vi "Drone.vi"() -> ()   [LabVIEW 2009]
uses:
  square.ctl
  Drone data.ctl
panel:
  out "iteration":i32
  in  "Import drones":path[](array[path])
  in  "create drones":T1[](array[typedef])=[{"Current"={"location"={"x"=0, "y"=0}, "checkpoint"=0}, "Checkpoints"=[{"x"=16, "y"=16}, {"x"=0, "y"=0}], "Color"=11145540, "Navigation style"=4}, {"Current"={"location"={"x"=31, "y"=16}, "checkpoint"=0}, "Checkpoints"=[{"x"=16, "y"=16}, {"x"=0, "y"=0}], "Color"=11145540, "Navigation style"=3}]
  in  "walls":path
  in  "stop":bool
  in  "Delay (ms)":u32
  out "map":T2[][](array[typedef])
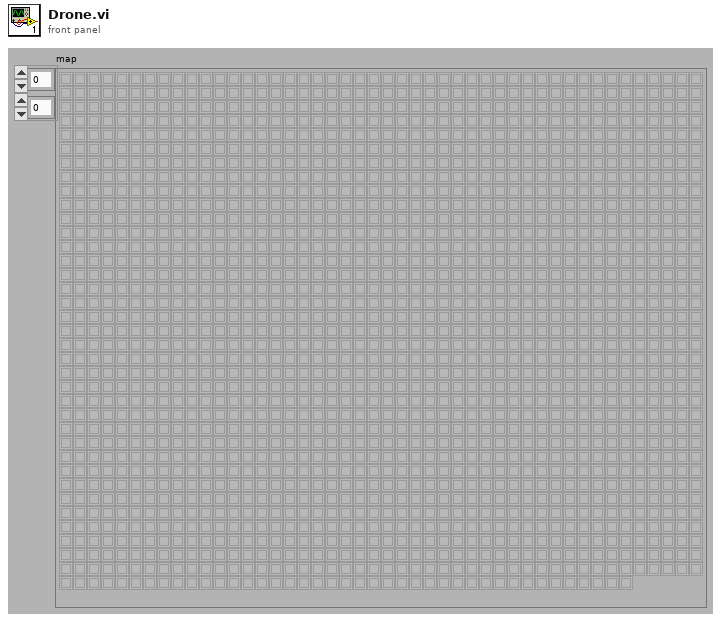
[diagram p1: front panel]
types:
  T1 = typedef "Drone data.ctl" = cluster{"Current":cluster{"location":cluster{"x":i16, "y":i16}, "checkpoint":i32}, "Checkpoints":cluster{"x":i16, "y":i16}[], "Color":u32, "Navigation style":i32}
  T2 = typedef "square.ctl" = u8
  T3 = typedef "direction.ctl" = i8
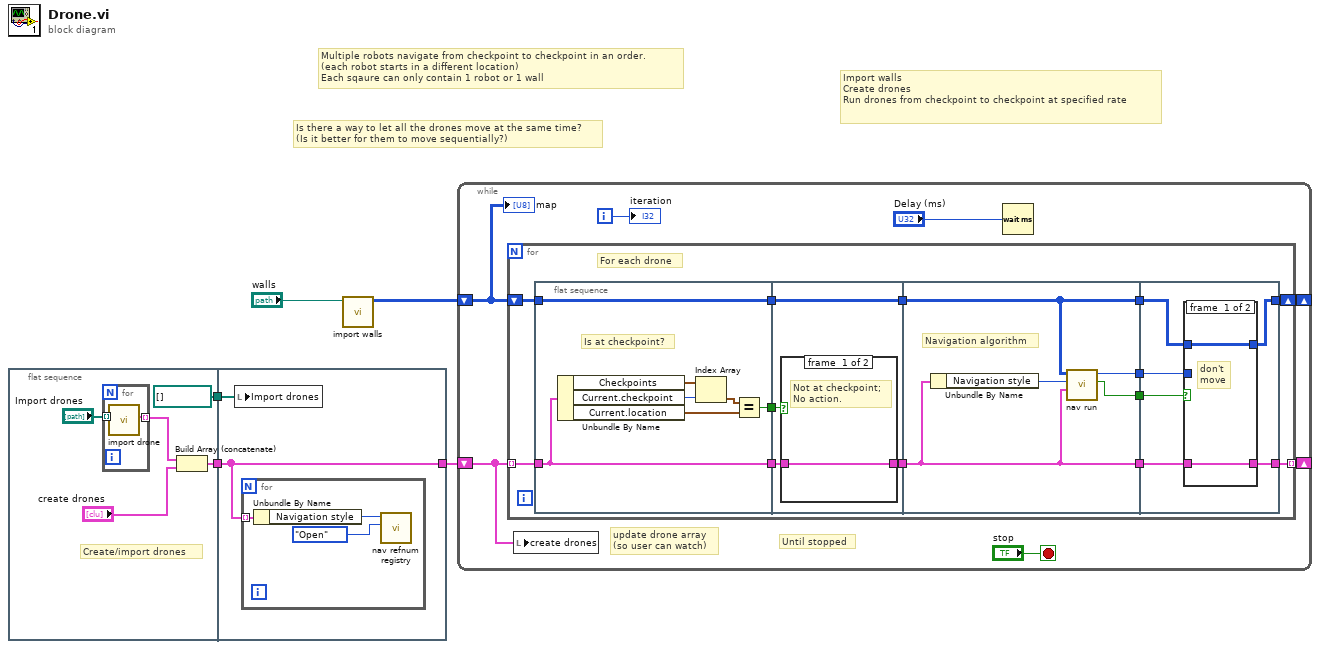
[diagram p0: block diagram]
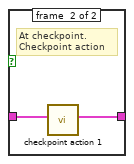
[diagram p2: hidden frame]
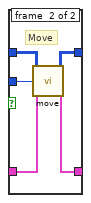
[diagram p3: hidden frame]
diagram:
  # "Is there a way to let all the drones move at the same time?\n(Is it better for them to move sequentially?)"
  # "Import walls\nCreate drones\nRun drones from checkpoint to checkpoint at specified rate"
  # "Multiple robots navigate from checkpoint to checkpoint in an order.\n(each robot starts in a different location)\nEach sqaure can only contain 1 robot or 1 wall"
  n1 = flat-sequence {
    tunnel: [w8] -> w2
    tunnel: [path[] [] ("Import drones")] -> w1
    tunnel: [w13] -> w3
    tunnel: w2 -> [w13]
    tunnel: w1 -> [w14]
    frame #0 {
      # "Create/import drones"
      n2 = for {
        tunnel: [w12] -> w10 mode=indexing
        tunnel: "Import drones" -> [w11] mode=indexing
        n3 = call "import drone.vi"("drone filepath"=w11) -> ("Drone"=w12:T1)  [unwired: 9 in, 1 out]
      }
      n4 = Build Array (concatenate)(w10, "create drones") -> (w8:T1[])
    }
    frame #1 {
      n5 = local write "Import drones"(w14) -> ()
      n6 = for {
        tunnel: w13 -> [w17] mode=indexing
        n7 = Unbundle By Name(w17) -> ("Navigation style"=w16:i32)
        n8 = call "nav refnum registry.vi"("Action"=enum16{"Open", "Retreive", "Close"}."Open", "nav type"=w16) -> ()  [unwired: 8 in, 2 out]
      }
    }
  }
  n9 = call "import walls.vi"("Picture path"="walls") -> ("walls/field"=w4:T2[][])  [unwired: 10 in]
  n10 = while {
    shift-right: [w24] -> _
    shift-left: w3 -> [w19]
    shift-right: [w23] -> _
    shift-left: w4 -> [w22]
    i -> [w18]
    stop <- "stop" stop-if-true
    # "update drone array\n(so user can watch)"
    # "Until stopped"
    n11 = for {
      tunnel: w19 -> [w36] mode=indexing
      tunnel: [w35] -> w24 mode=indexing
      shift-right: [w30] -> w23
      shift-left: w22 -> [w27]
      # "For each drone"
      n12 = flat-sequence {
        tunnel: [w39] -> w37
        tunnel: w36 -> [w38]
        tunnel: [w38] -> w32
        tunnel: [w44] -> w28
        tunnel: w27 -> [w44]
        tunnel: w37 -> [w48]
        tunnel: [w46] -> w33
        tunnel: w32 -> [w45]
        tunnel: [w47] -> w29
        tunnel: w28 -> [w47]
        tunnel: [w54] -> w34
        tunnel: [w55] -> w31
        tunnel: w29 -> [w55]
        tunnel: w33 -> [w54]
        tunnel: [w53] -> w26
        tunnel: [w52] -> w25
        tunnel: [w60] -> w35
        tunnel: w34 -> [w59]
        tunnel: [w61] -> w30
        tunnel: w31 -> [w62]
        tunnel: w26 -> [w58]
        tunnel: w25 -> [w57]
        frame #0 {
          # "Is at checkpoint?"
          n13 = Unbundle By Name(w38) -> ("Checkpoints"=w42:cluster{"x":i16, "y":i16}[], "Current.checkpoint"=w43:i32, "Current.location"=w40:cluster{"x":i16, "y":i16})
          n14 = Index Array(array=w42, index=w43) -> (element=w41:cluster{"x":i16, "y":i16})
          n15 = Equal?(x=w41, y=w40) -> (x = y?=w39:bool)
        }
        frame #1 {
          n16 = case shown="True" w48 {
            tunnel: [w49 w50] -> w46
            tunnel: w45 -> [w49 w51]
            frame #0 {
              # "Not at checkpoint;\nNo action."
            }
            frame #1 {
              # "At checkpoint.\nCheckpoint action"
              n17 = call "checkpoint action 1.vi"("Drone"=w51) -> ("Drone"=w50:T1)  [unwired: 10 in]
            }
          }
        }
        frame #2 {
          # "Navigation algorithm"
          n18 = Unbundle By Name(w54) -> ("Navigation style"=w56:i32)
          n19 = call "nav run.vi"("Drone"=w54, "nav type"=w56, "Field"=w55) -> ("Move?"=w52:bool, "direction"=w53:T3)  [unwired: 7 in]
        }
        frame #3 {
          n20 = case shown="True" w57 {
            tunnel: w62 -> [w64 w69]
            tunnel: [w64 w67] -> w61
            tunnel: [w63 w66] -> w60
            tunnel: w59 -> [w63 w68]
            tunnel: w58 -> [_ w65]
            frame #0 {
              # "don't\nmove"
            }
            frame #1 {
              # "Move"
              n21 = call "move.vi"("walls/field"=w69, "direction"=w65, "Drone"=w68) -> ("walls/field"=w67:T2[][], "Drone"=w66:T1)  [unwired: 5 in]
            }
          }
        }
      }
    }
    n22 = local write "create drones"(w19) -> ()
    n23 = Wait (ms)(milliseconds to wait="Delay (ms)") -> ()  [unwired: 1 out]
    "map" <- w22
    "iteration" <- w18
  }
